vi "exec.vi"(8 "error in (no error)":errorcluster, 11 "ChangeSlitWidth in":refnum<class "ChangeSlitWidth.lvclass">) -> (0 "error out":errorcluster, 3 "ChangeSlitWidth out":refnum<class "ChangeSlitWidth.lvclass">)   [LabVIEW 2016, in "ChangeSlitWidth.lvclass"]
uses:
  ChangeSlitWidth.lvclass
  C:/Users/aanania/Documents/ts_monochromator_windows/WindowsController/Commands/Command/Command.lvclass
  Command/Command.lvclass/Command.ctl
  ChangeSlitWidth.lvclass/ChangeSlitWidth.ctl
  Command/Command.lvclass
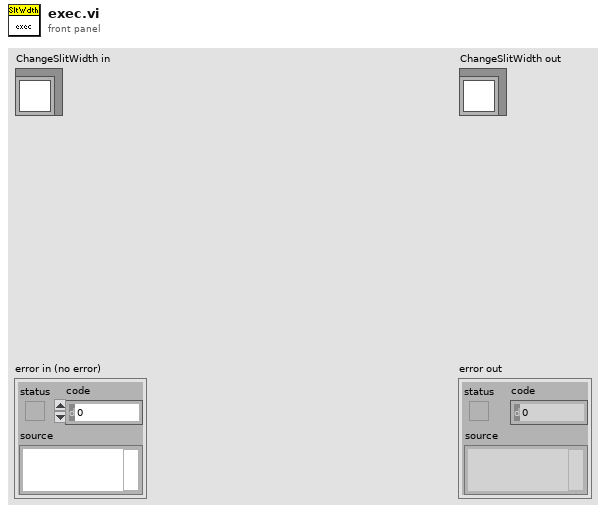
[diagram p1: front panel]
types:
  T1 = typedef "SlitType.ctl" = enum16{"Front Entrance", "Side Entrance", "Front Exit", "Side Exit", "First Intermediate", "Second Intermediate"}
  T2 = typedef "slitWidth.ctl" = dbl
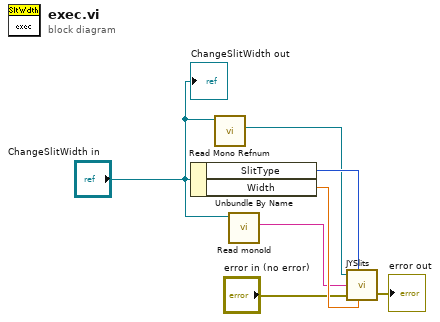
[diagram p0: block diagram]
diagram:
  n1 = Unbundle By Name("ChangeSlitWidth in") -> ("SlitType"=w6:T1, "Width"=w7:T2)
  n2 = call "Read Mono Refnum.vi"("Command in"="ChangeSlitWidth in") -> ("Mono Refnum"=w1:refnum<k7>)  [unwired: 8 in, 2 out]
  n3 = call "Read monoId.vi"("Command in"="ChangeSlitWidth in") -> ("monoId"=w2:string)  [unwired: 8 in, 2 out]
  n4 = call "JYSlits.vi"("JYMONOLib.IJYMonoReqd"=w1, "Slit"=w6, "UniqueID"=w2, "error in (no error)"="error in (no error)", "Slit Width"=w7) -> ("error out"=→"error out":errorcluster)  [unwired: 1 out]
  "ChangeSlitWidth out" <- "ChangeSlitWidth in"
